vi "(SubVI) Stage WritePI.vi"(3 "axis":u32, 5 "position":dbl) -> ()   [LabVIEW 2014]
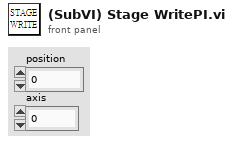
[diagram p1: front panel]
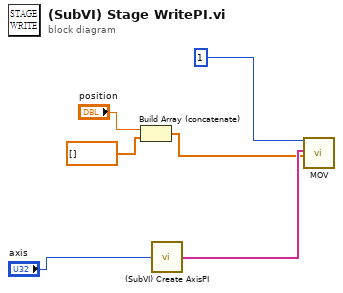
[diagram p0: block diagram]
diagram:
  n1 = Build Array (concatenate)("position", dbl[] []) -> (w1:dbl[])
  n2 = call "(SubVI) Create AxisPI.vi"("axis"="axis") -> ("Array"=w4:string[])  [unwired: 4 in]
  n3 = call "MOV.vi"("System no."=1, "Axes to move"=w4, "Position values"=w1) -> ()  [unwired: 16 in, 1 out]
